vi "Regenerate Split Nodes Tag.vi"(7 "Tree In":refnum<class "Tree.lvclass">, 9 "Start Index":i32, 10 "Split Node In":refnum<class "Tree Data.lvclass">[](array[class]), 11 "Parent Tag In":string) -> (2 "Split Node Out":refnum<class "Tree Data.lvclass">[](array[class]), 3 "Parent Tag Out":string, 5 "Tree Out":refnum<class "Tree.lvclass">)   [LabVIEW 2024, in "Composite Tree Data.lvclass"]
uses:
  Composite Tree Data.lvclass
  Tree Data/Tree Data.lvclass
  Tree/Tree.lvclass
  Tree Data/Tree Data.lvclass/Tree Data.ctl
  Tree Data/Protected Data/Read Tag.vi
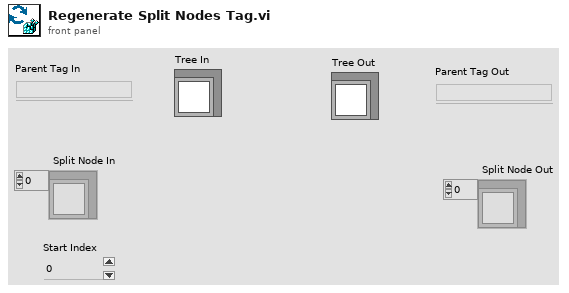
[diagram p1: front panel]
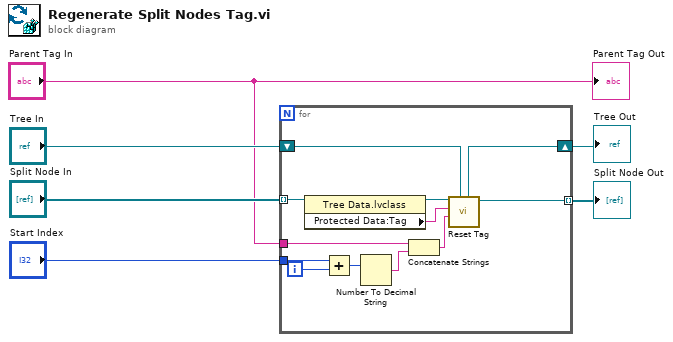
[diagram p0: block diagram]
diagram:
  n1 = for {
    tunnel: "Split Node In" -> [w18] mode=indexing
    tunnel: [w16] -> w5 mode=indexing
    shift-right: [w14] -> w3
    shift-left: "Tree In" -> [w15]
    tunnel: "Parent Tag In" -> [w8]
    tunnel: "Start Index" -> [w11]
    i -> [w12]
    n2 = property class="Tree Data.lvclass"(reference=w18) -> (reference out=w17:refnum<class "Tree Data.lvclass">, "Protected Data:Tag"=w13:string)  [unwired: 1 in, 1 out]
    n3 = Add(x=w11, y=w12) -> (x+y=w10:i32)
    n4 = Number To Decimal String(number=w10) -> (decimal integer string=w9:string)  [unwired: 1 in]
    n5 = Concatenate Strings(w8, w9) -> (w7:string)
    n6 = call-dynamic "Reset Tag.vi"("Tree In"=w15, "New Tag"=w7, "Original Tag"=w13, "Tree Data in"=w17) -> ("Tree Data out"=w16:refnum<class "Tree Data.lvclass">, "Tree Out"=w14:refnum<class "Tree.lvclass">)  [unwired: 5 in, 1 out]
  }
  "Split Node Out" <- w5
  "Tree Out" <- w3
  "Parent Tag Out" <- "Parent Tag In"
